vi "FisherPaykel Agitate State.vi"(0 "VISA Refnum in":refnum<visa-resource-name>, 1 "Debug":bool, 2 "Use GEA Inverter Output":bool, 5 "Agitate Parameters":T3 {"PauseTime (0-1800ms 10ms Increment)" step=10; "PlateauTime (0-1800ms 10ms Increment)" step=10; "TargetSpeed (0-200RPM)" max=1600 step=1; "RampUpTime (1-600ms)" max=600 step=10; "Agitate Running Time (sec)" step=1}, 7 "GEA2 Reference In":refnum<k24>, 11 "Error In":errorcluster, 12 "Agitate PID":T2={"Kp"=1.84, "Ki"=0.03, "Kd"=0.0, "Kc"=0.06} {"Kc" min=0.0 max=1.0; "Kd" min=0.0 max=1.0; "Ki" min=0.0 max=1.0; "Kp" min=0.0 max=16.0}, 13 "Agitate CMD Speed":u32=150, 14 "GEA Inputs":T1={"Source"=228, "Destination"=35} {"Destination" format="%.0x"; "Source" format="%.0x"}) -> (4 "VISA resource name out":refnum<visa-resource-name>, 8 "GEA2 Reference Out":refnum<k24>, 15 "Error Out":errorcluster)   [LabVIEW 2016]
uses:
  Type Definitions/Fisher Paykel Agitate Parameters.ctl
  Type Definitions/FisherPaykel Direction CMD.ctl
  Type Definitions/Fisher Paykel Spin PID.ctl
  C:/Technology Lab/NI-2010/Trunk/Utility/LabVIEW GEA2 Toolkit v1.0.0.0/Appliance.NET/GeaCommunication.dll
  Trunk/Utility/LabVIEW GEA2 Toolkit v1.0.0.0/Appliance.NET/GeaCommunication.dll
  Trunk/Utility/LabVIEW GEA2 Toolkit v1.0.0.0/type defs/Source_Destination.ctl
  Type Definitions/Fisher Paykel Main Command.ctl
  Trunk/Utility/LabVIEW GEA2 Toolkit v1.0.0.0/library/GEA2_Toolkit.lvlib
panel:
  # "Agitate Profile Parameters"
  # "Agitate Start Parameters"
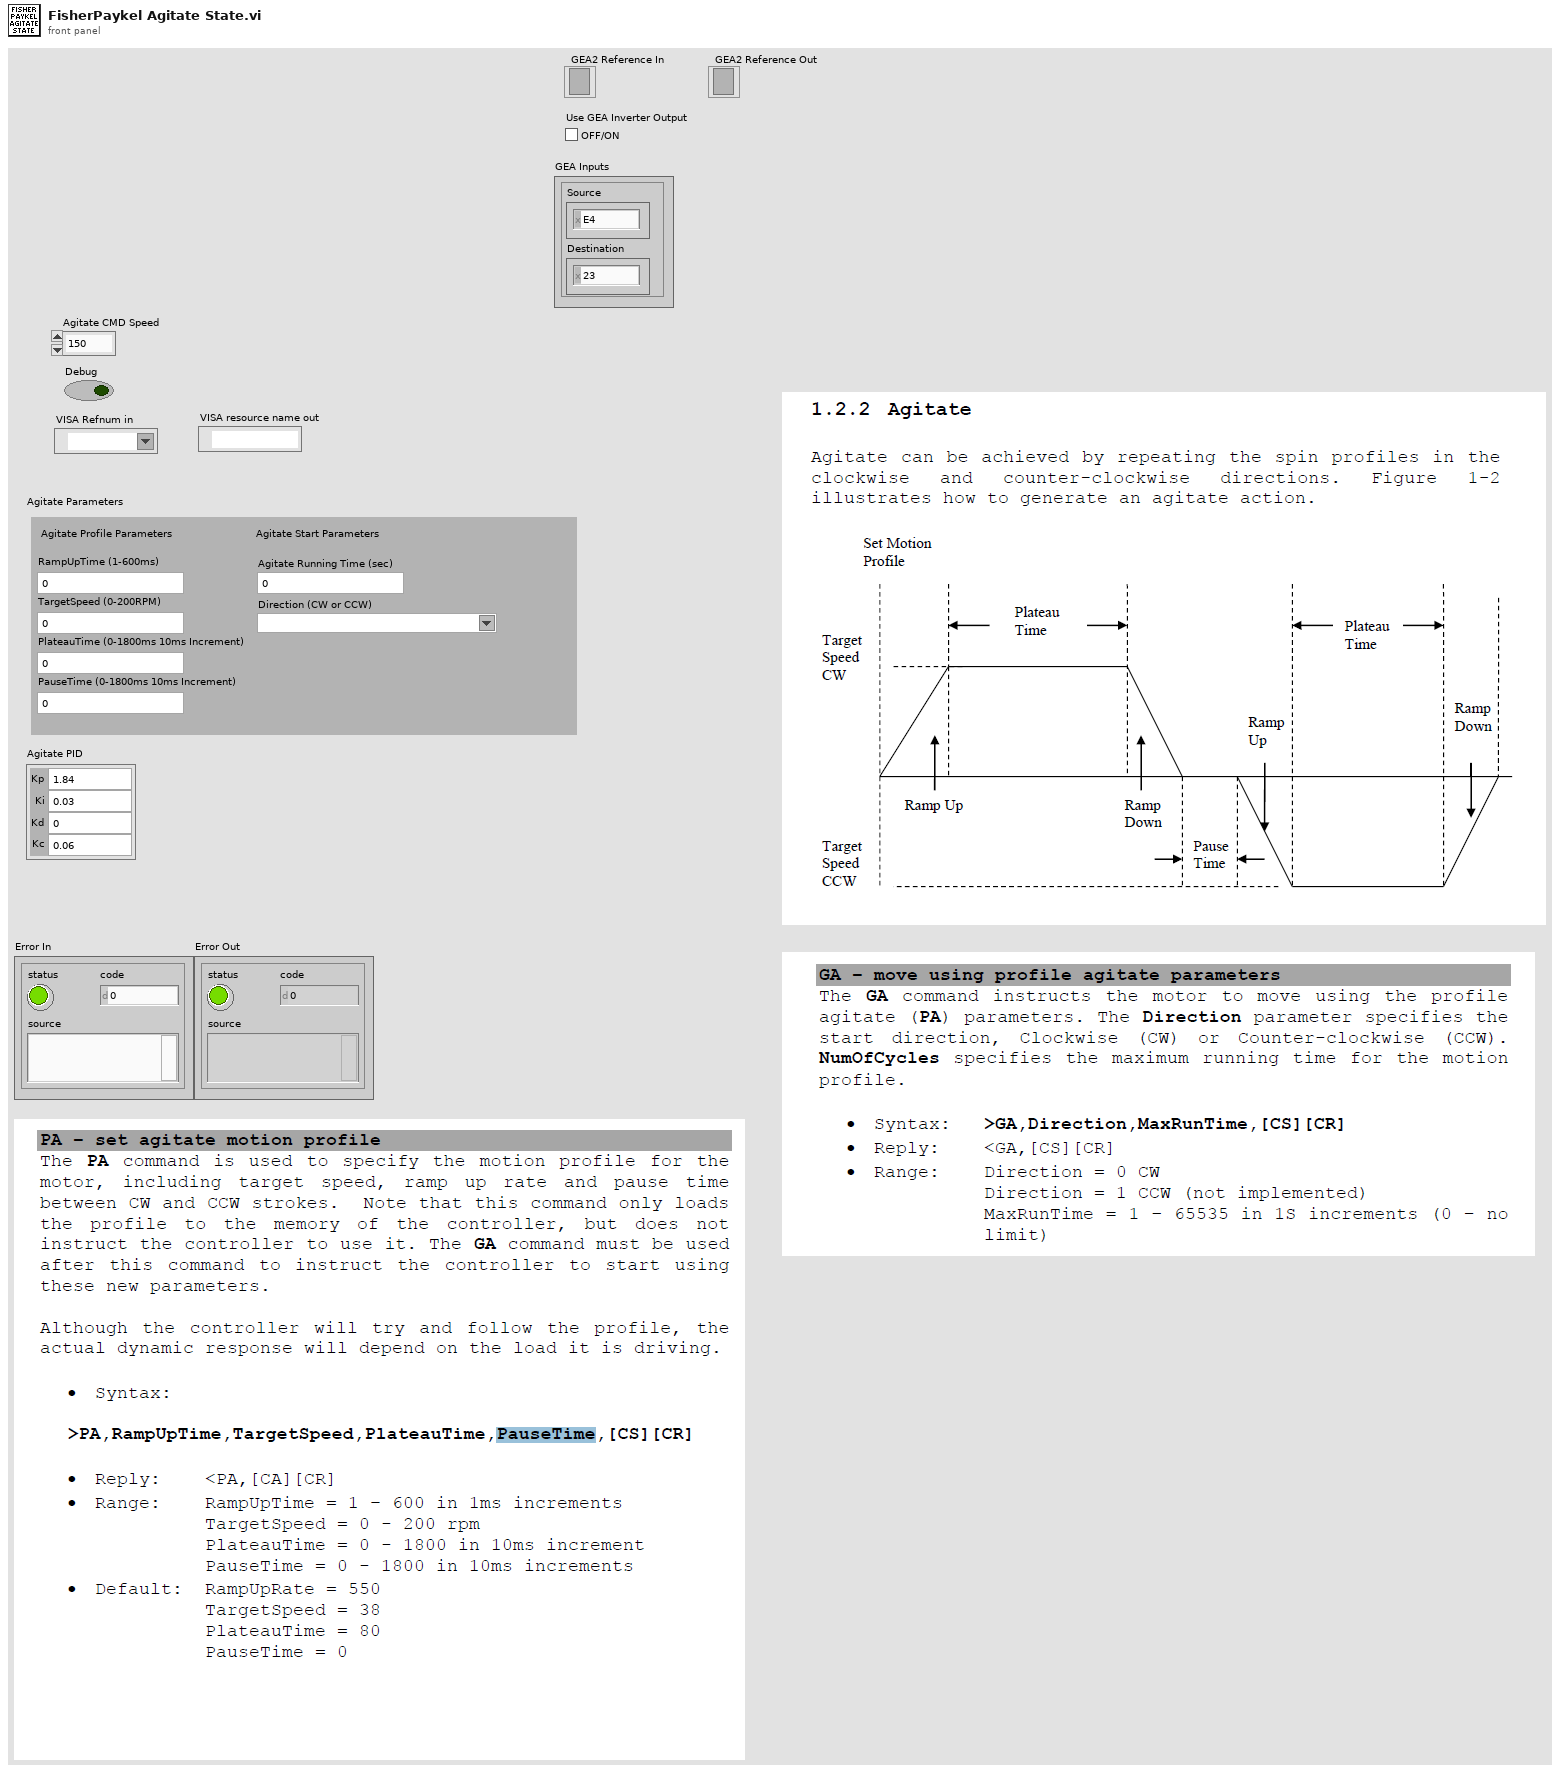
[diagram p1: front panel]
types:
  T1 = typedef "GEA2_Toolkit.lvlib/Source_Destination.ctl" = cluster{"Source":u8, "Destination":u8}
  T2 = typedef "Fisher Paykel Spin PID.ctl" = cluster{"Kp":dbl, "Ki":dbl, "Kd":dbl, "Kc":dbl}
  T3 = typedef "Fisher Paykel Agitate Parameters.ctl" = cluster{"Agitate Running Time (sec)":u16, "Direction (CW or CCW)":T4, "RampUpTime (1-600ms)":u16, "TargetSpeed (0-200RPM)":u16, "PlateauTime (0-1800ms 10ms Increment)":u16, "PauseTime (0-1800ms 10ms Increment)":u16}
  T4 = typedef "FisherPaykel Direction CMD.ctl" = string
  T5 = typedef "Fisher Paykel Main Command.ctl" = string
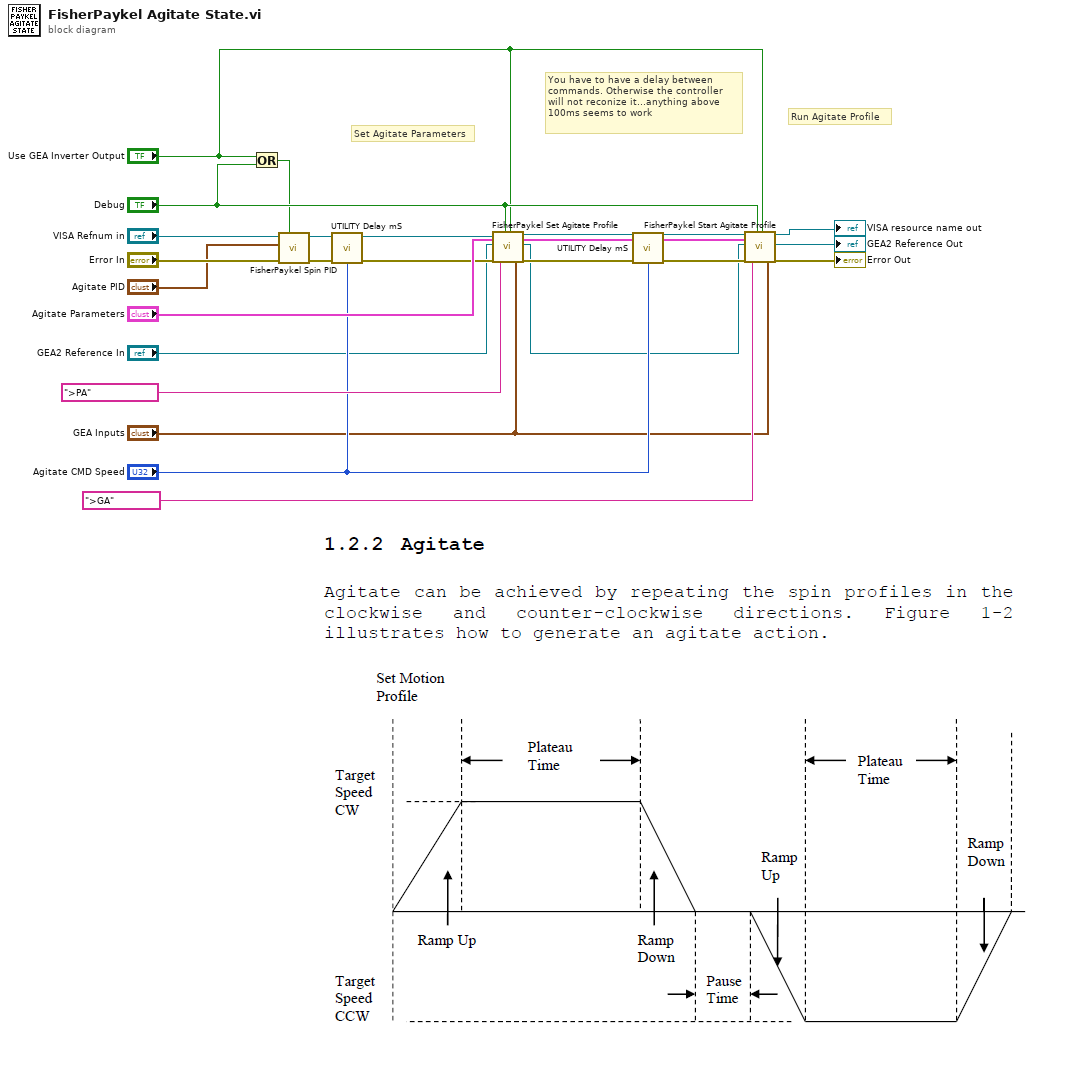
[diagram p0: block diagram]
diagram:
  # "You have to have a delay between \ncommands. Otherwise the controller\nwill not reconize it...anything above\n100ms seems to work"
  # "Run Agitate Profile"
  # "Set Agitate Parameters"
  n1 = Or(x="Use GEA Inverter Output", y="Debug") -> (x .or. y?=w6:bool)
  n2 = call "FisherPaykel Spin PID.vi"("Debug"=w6, "Error In"="Error In", "Spin PID"="Agitate PID", "VISA Refnum in"="VISA Refnum in") -> ("Error Out"=w14:errorcluster, "VISA Refnum out"=w10:refnum<visa-resource-name>)  [unwired: 6 in]
  n3 = call "UTILITY Delay mS.vi"("Error In"=w14, "milliseconds to wait"="Agitate CMD Speed") -> ("Error Out"=w12:errorcluster)  [unwired: 13 in]
  n4 = call "FisherPaykel Set Agitate Profile.vi"("VISA Refnum in"=w10, "Agitate Parameters"="Agitate Parameters", "GEA2 Reference In"="GEA2 Reference In", "Error In"=w12, "Main Command"=T5 ">PA", "Debug"="Debug", "Use GEA Inverter Output"="Use GEA Inverter Output", "GEA Inputs"="GEA Inputs") -> ("VISA resource name out"=w19:refnum<visa-resource-name>, "Agitate Parameters Out"=w15:T3, "GEA2 Reference Out"=w3:refnum<k24>, "Error Out"=w22:errorcluster)  [unwired: 8 in]
  n5 = call "UTILITY Delay mS.vi"("Error In"=w22, "milliseconds to wait"="Agitate CMD Speed") -> ("Error Out"=w21:errorcluster)  [unwired: 13 in]
  n6 = call "FisherPaykel Start Agitate Profile.vi"("VISA Refnum in"=w19, "Agitate Parameters"=w15, "GEA2 Reference In"=w3, "Error In"=w21, "Main Command"=T5 ">GA" ("Main Command 2"), "Debug"="Debug", "Use GEA Inverter Output"="Use GEA Inverter Output", "GEA Inputs"="GEA Inputs") -> ("VISA resource name out"=→"VISA resource name out":refnum<visa-resource-name>, "GEA2 Reference Out"=→"GEA2 Reference Out":refnum<k24>, "Error Out"=→"Error Out":errorcluster)  [unwired: 9 in]
